vi "supervision.vi"() -> ()   [LabVIEW 2015]
uses:
  <vilib>/httpClient/LabVIEWHTTPClient.lvlib
panel:
  out "body":string
  in  "OK Button 8":bool
  out "Luminosité Séjour":dbl(knob) scale=0.0..100.0
  out "Luminosité Cuisine":dbl(knob) scale=0.0..100.0
  out "Luminosité Salon":dbl(knob) scale=0.0..100.0
  out "Humidité Cuisine":dbl(slide) scale=0.0..100.0
  out "Humidité Salon":dbl(slide) scale=0.0..100.0
  out "Humidité Séjour":dbl(slide) scale=0.0..100.0
  out "Température Séjour":dbl(slide) scale=0.0..40.0
  out "Température Cuisine":dbl(slide) scale=0.0..40.0
  out "Température Salon":dbl(slide) scale=0.0..40.0
  out "ENERGIE":dbl(graph)
  out "GAZ":dbl(graph)
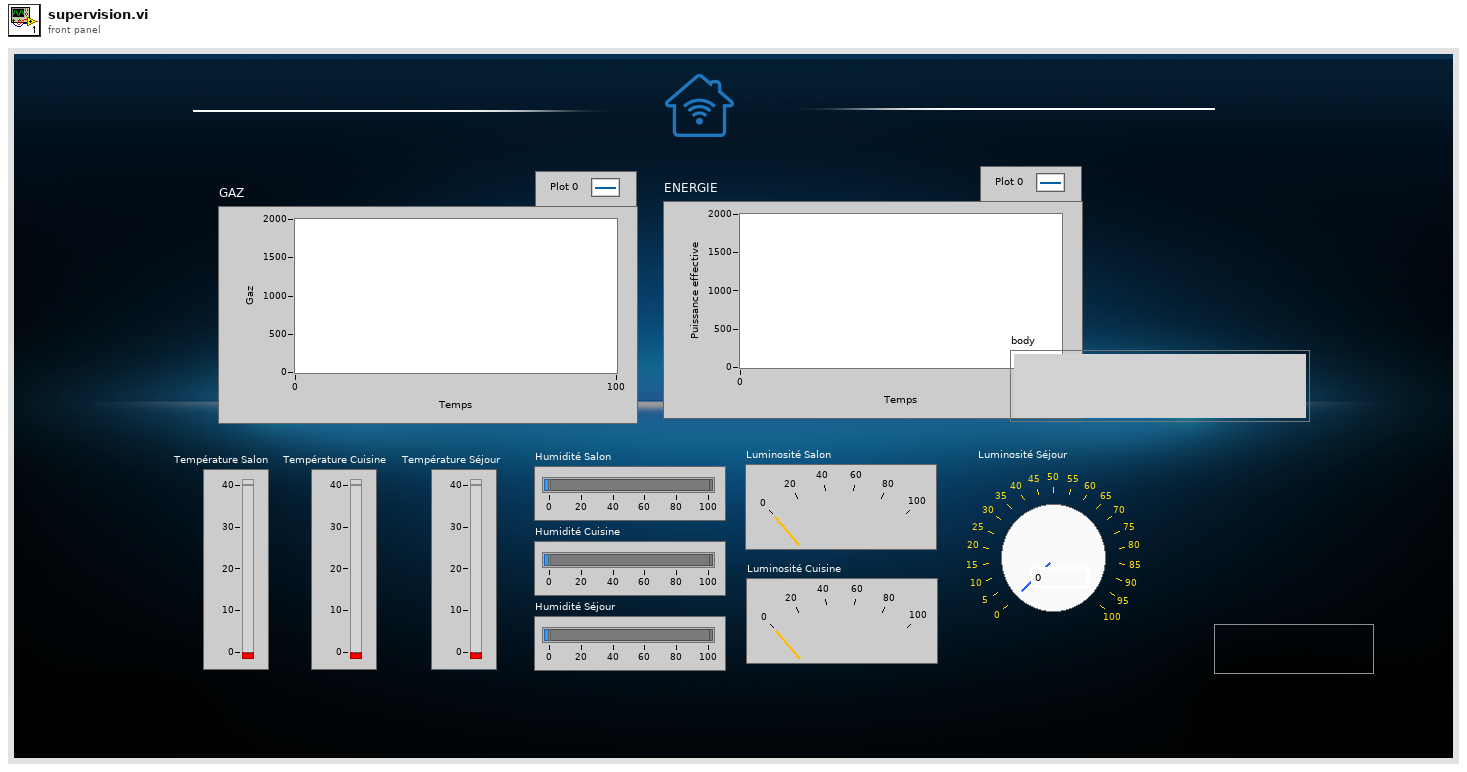
[diagram p1: front panel]
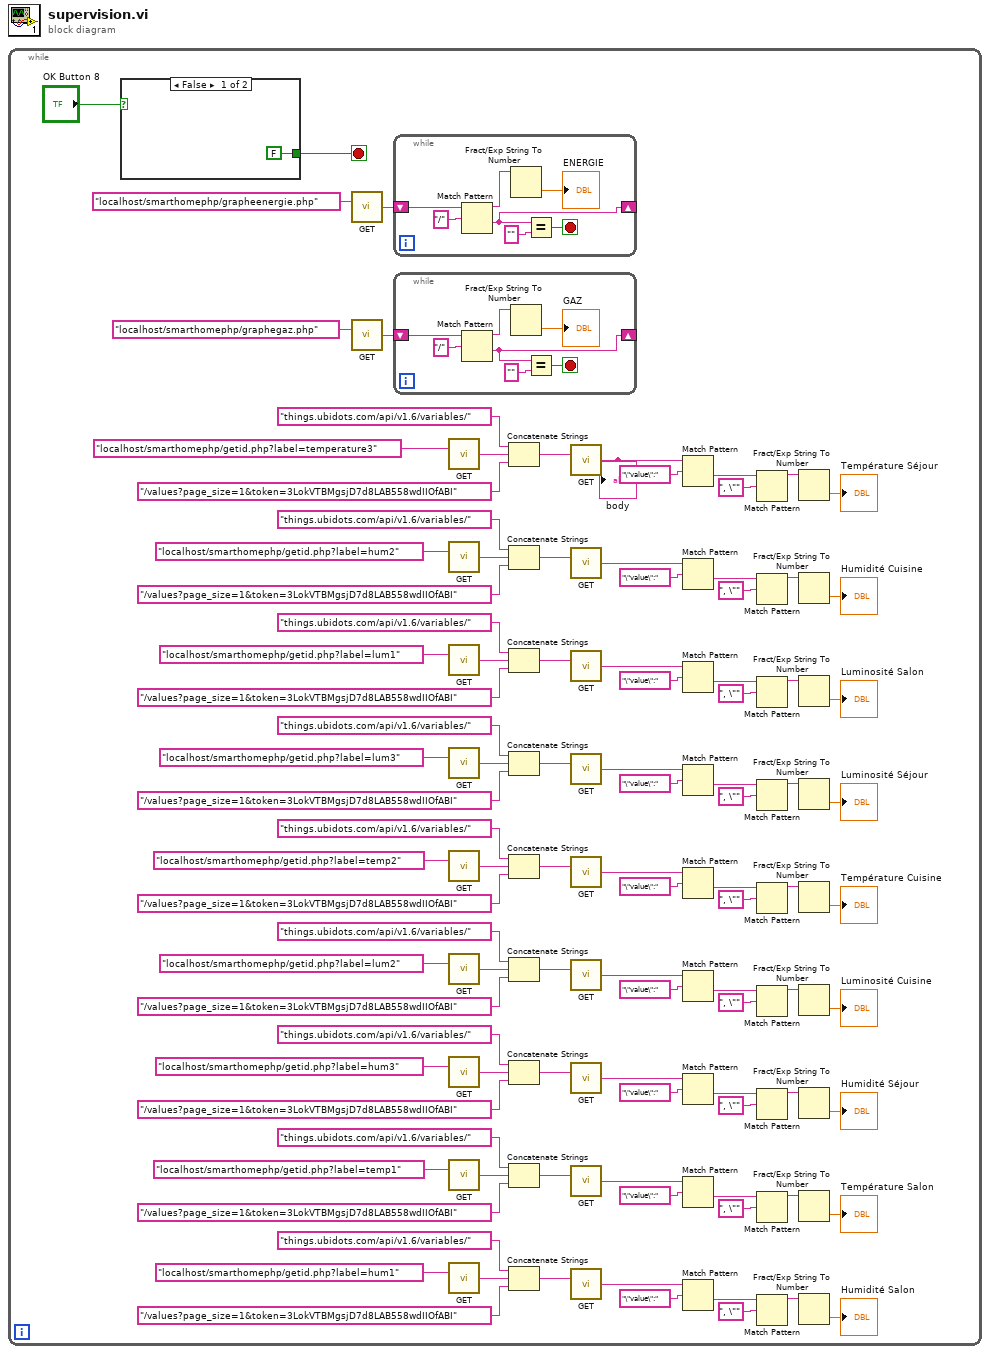
[diagram p0: block diagram]
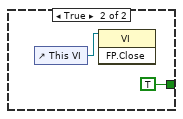
[diagram p2: hidden frame]
diagram:
  n1 = while {
    stop <- w102 stop-if-true
    n2 = case shown="False" "OK Button 8" {
      tunnel: [FALSE TRUE] -> w102
      frame False {
      }
      frame True {
        n3 = control-ref of="This VI"() -> (w115:refnum<vi>)
        n4 = invoke class="VI" method="FP.Close"(reference=w115) -> ()  [unwired: 2 in, 3 out]
      }
    }
    n5 = call <vilib>:"GET.vi"("url"="localhost/smarthomephp/grapheenergie.php") -> ("body"=w104:string)  [unwired: 11 in, 3 out]
    n6 = call <vilib>:"GET.vi"("url"="localhost/smarthomephp/graphegaz.php") -> ("body"=w46:string)  [unwired: 11 in, 3 out]
    n7 = while {
      shift-right: [w118] -> _
      shift-left: w104 -> [w121]
      stop <- w116 stop-if-true
      n8 = Match Pattern(string=w121, regular expression="/") -> (before substring=w120:string, after substring=w118:string)  [unwired: 1 in, 2 out]
      n9 = Fract/Exp String To Number(string=w120) -> (number=→"ENERGIE":dbl)  [unwired: 3 in, 1 out]
      n10 = Equal?(x=w118, y="") -> (x = y?=w116:bool)
    }
    n11 = while {
      shift-right: [w109] -> _
      shift-left: w46 -> [w111]
      stop <- w107 stop-if-true
      n12 = Match Pattern(string=w111, regular expression="/") -> (before substring=w110:string, after substring=w109:string)  [unwired: 1 in, 2 out]
      n13 = Fract/Exp String To Number(string=w110) -> (number=→"GAZ":dbl)  [unwired: 3 in, 1 out]
      n14 = Equal?(x=w109, y="") -> (x = y?=w107:bool)
    }
    n15 = call <vilib>:"GET.vi"("url"="localhost/smarthomephp/getid.php?label=temperature3") -> ("body"=w6:string)  [unwired: 11 in, 3 out]
    n16 = call <vilib>:"GET.vi"("url"="localhost/smarthomephp/getid.php?label=hum2") -> ("body"=w23:string)  [unwired: 11 in, 3 out]
    n17 = call <vilib>:"GET.vi"("url"="localhost/smarthomephp/getid.php?label=lum1") -> ("body"=w25:string)  [unwired: 11 in, 3 out]
    n18 = call <vilib>:"GET.vi"("url"="localhost/smarthomephp/getid.php?label=lum3") -> ("body"=w44:string)  [unwired: 11 in, 3 out]
    n19 = call <vilib>:"GET.vi"("url"="localhost/smarthomephp/getid.php?label=temp2") -> ("body"=w48:string)  [unwired: 11 in, 3 out]
    n20 = call <vilib>:"GET.vi"("url"="localhost/smarthomephp/getid.php?label=lum2") -> ("body"=w67:string)  [unwired: 11 in, 3 out]
    n21 = call <vilib>:"GET.vi"("url"="localhost/smarthomephp/getid.php?label=hum3") -> ("body"=w71:string)  [unwired: 11 in, 3 out]
    n22 = call <vilib>:"GET.vi"("url"="localhost/smarthomephp/getid.php?label=temp1") -> ("body"=w89:string)  [unwired: 11 in, 3 out]
    n23 = call <vilib>:"GET.vi"("url"="localhost/smarthomephp/getid.php?label=hum1") -> ("body"=w93:string)  [unwired: 11 in, 3 out]
    n24 = Concatenate Strings("things.ubidots.com/api/v1.6/variables/", w6, "/values?page_size=1&token=3LokVTBMgsjD7d8LAB558wdIIOfABI" ("string")) -> (w8:string)
    n25 = Concatenate Strings("things.ubidots.com/api/v1.6/variables/", w23, "/values?page_size=1&token=3LokVTBMgsjD7d8LAB558wdIIOfABI" ("string")) -> (w21:string)
    n26 = Concatenate Strings("things.ubidots.com/api/v1.6/variables/", w25, "/values?page_size=1&token=3LokVTBMgsjD7d8LAB558wdIIOfABI" ("string")) -> (w27:string)
    n27 = Concatenate Strings("things.ubidots.com/api/v1.6/variables/", w44, "/values?page_size=1&token=3LokVTBMgsjD7d8LAB558wdIIOfABI" ("string")) -> (w41:string)
    n28 = Concatenate Strings("things.ubidots.com/api/v1.6/variables/", w48, "/values?page_size=1&token=3LokVTBMgsjD7d8LAB558wdIIOfABI" ("string")) -> (w51:string)
    n29 = Concatenate Strings("things.ubidots.com/api/v1.6/variables/", w67, "/values?page_size=1&token=3LokVTBMgsjD7d8LAB558wdIIOfABI" ("string")) -> (w65:string)
    n30 = Concatenate Strings("things.ubidots.com/api/v1.6/variables/", w71, "/values?page_size=1&token=3LokVTBMgsjD7d8LAB558wdIIOfABI" ("string")) -> (w73:string)
    n31 = Concatenate Strings("things.ubidots.com/api/v1.6/variables/", w89, "/values?page_size=1&token=3LokVTBMgsjD7d8LAB558wdIIOfABI" ("string")) -> (w87:string)
    n32 = Concatenate Strings("things.ubidots.com/api/v1.6/variables/", w93, "/values?page_size=1&token=3LokVTBMgsjD7d8LAB558wdIIOfABI" ("string")) -> (w95:string)
    n33 = call <vilib>:"GET.vi"("url"=w8) -> ("body"=w9:string)  [unwired: 11 in, 3 out]
    "body" <- w9
    n34 = call <vilib>:"GET.vi"("url"=w21) -> ("body"=w20:string)  [unwired: 11 in, 3 out]
    n35 = call <vilib>:"GET.vi"("url"=w27) -> ("body"=w28:string)  [unwired: 11 in, 3 out]
    n36 = call <vilib>:"GET.vi"("url"=w41) -> ("body"=w40:string)  [unwired: 11 in, 3 out]
    n37 = call <vilib>:"GET.vi"("url"=w51) -> ("body"=w52:string)  [unwired: 11 in, 3 out]
    n38 = call <vilib>:"GET.vi"("url"=w65) -> ("body"=w64:string)  [unwired: 11 in, 3 out]
    n39 = call <vilib>:"GET.vi"("url"=w73) -> ("body"=w74:string)  [unwired: 11 in, 3 out]
    n40 = call <vilib>:"GET.vi"("url"=w87) -> ("body"=w86:string)  [unwired: 11 in, 3 out]
    n41 = call <vilib>:"GET.vi"("url"=w95) -> ("body"=w96:string)  [unwired: 11 in, 3 out]
    n42 = Match Pattern(string=w9, regular expression="\"value\":") -> (after substring=w11:string)  [unwired: 1 in, 3 out]
    n43 = Match Pattern(string=w20, regular expression="\"value\":") -> (after substring=w18:string)  [unwired: 1 in, 3 out]
    n44 = Match Pattern(string=w28, regular expression="\"value\":") -> (after substring=w30:string)  [unwired: 1 in, 3 out]
    n45 = Match Pattern(string=w40, regular expression="\"value\":") -> (after substring=w38:string)  [unwired: 1 in, 3 out]
    n46 = Match Pattern(string=w52, regular expression="\"value\":") -> (after substring=w54:string)  [unwired: 1 in, 3 out]
    n47 = Match Pattern(string=w64, regular expression="\"value\":") -> (after substring=w62:string)  [unwired: 1 in, 3 out]
    n48 = Match Pattern(string=w74, regular expression="\"value\":") -> (after substring=w76:string)  [unwired: 1 in, 3 out]
    n49 = Match Pattern(string=w86, regular expression="\"value\":") -> (after substring=w84:string)  [unwired: 1 in, 3 out]
    n50 = Match Pattern(string=w96, regular expression="\"value\":") -> (after substring=w98:string)  [unwired: 1 in, 3 out]
    n51 = Match Pattern(string=w11, regular expression=", \"") -> (before substring=w13:string)  [unwired: 1 in, 3 out]
    n52 = Match Pattern(string=w18, regular expression=", \"") -> (before substring=w16:string)  [unwired: 1 in, 3 out]
    n53 = Match Pattern(string=w30, regular expression=", \"") -> (before substring=w32:string)  [unwired: 1 in, 3 out]
    n54 = Match Pattern(string=w38, regular expression=", \"") -> (before substring=w36:string)  [unwired: 1 in, 3 out]
    n55 = Match Pattern(string=w54, regular expression=", \"") -> (before substring=w56:string)  [unwired: 1 in, 3 out]
    n56 = Match Pattern(string=w62, regular expression=", \"") -> (before substring=w60:string)  [unwired: 1 in, 3 out]
    n57 = Match Pattern(string=w76, regular expression=", \"") -> (before substring=w78:string)  [unwired: 1 in, 3 out]
    n58 = Match Pattern(string=w84, regular expression=", \"") -> (before substring=w82:string)  [unwired: 1 in, 3 out]
    n59 = Match Pattern(string=w98, regular expression=", \"") -> (before substring=w100:string)  [unwired: 1 in, 3 out]
    n60 = Fract/Exp String To Number(string=w13) -> (number=→"Température Séjour":dbl)  [unwired: 3 in, 1 out]
    n61 = Fract/Exp String To Number(string=w16) -> (number=→"Humidité Cuisine":dbl)  [unwired: 3 in, 1 out]
    n62 = Fract/Exp String To Number(string=w32) -> (number=→"Luminosité Salon":dbl)  [unwired: 3 in, 1 out]
    n63 = Fract/Exp String To Number(string=w36) -> (number=→"Luminosité Séjour":dbl)  [unwired: 3 in, 1 out]
    n64 = Fract/Exp String To Number(string=w56) -> (number=→"Température Cuisine":dbl)  [unwired: 3 in, 1 out]
    n65 = Fract/Exp String To Number(string=w60) -> (number=→"Luminosité Cuisine":dbl)  [unwired: 3 in, 1 out]
    n66 = Fract/Exp String To Number(string=w78) -> (number=→"Humidité Séjour":dbl)  [unwired: 3 in, 1 out]
    n67 = Fract/Exp String To Number(string=w82) -> (number=→"Température Salon":dbl)  [unwired: 3 in, 1 out]
    n68 = Fract/Exp String To Number(string=w100) -> (number=→"Humidité Salon":dbl)  [unwired: 3 in, 1 out]
  }
